vi "GOOP_CreateDefaultIniFile.vi"() -> (1 "NativeRead":path, 2 "NativeWrite":path)   [LabVIEW 2020]
uses:
  <resource>/Framework/Providers/Open_GDS/ClassProviders/Provider_EndevoGOOP300/EndevoProviderName.ctl
  <resource>/Framework/Providers/Open_GDS/ClassProviders/Provider_LvNativeClass/LvNativeProviderName.ctl
  <resource>/Framework/Providers/Open_GDS/ClassProviders/Provider_EndevoGOOP400/EndevoG4ProviderName.ctl
  <vilib>/Utility/config.llb/Write Key (String).vi
  <vilib>/Utility/config.llb/NI_LVConfig.lvlib
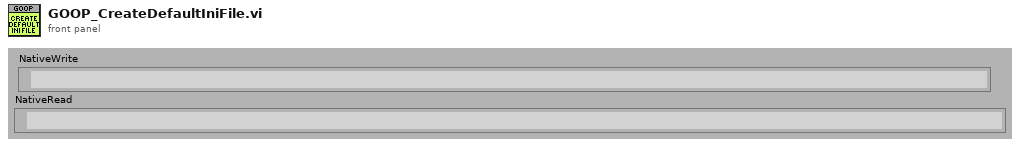
[diagram p1: front panel]
types:
  T1 = typedef "EndevoG4ProviderName.ctl" = enum16{"EndevoGOOP400"}
  T2 = typedef "LvNativeProviderName.ctl" = enum16{"Endevo LabVIEW Native"}
  T3 = typedef "EndevoProviderName.ctl" = enum16{"EndevoGOOP300"}
  T4 = typedef "NI_LVConfig.lvlib/Config Data RefNum.ctl" = refnum<k1>
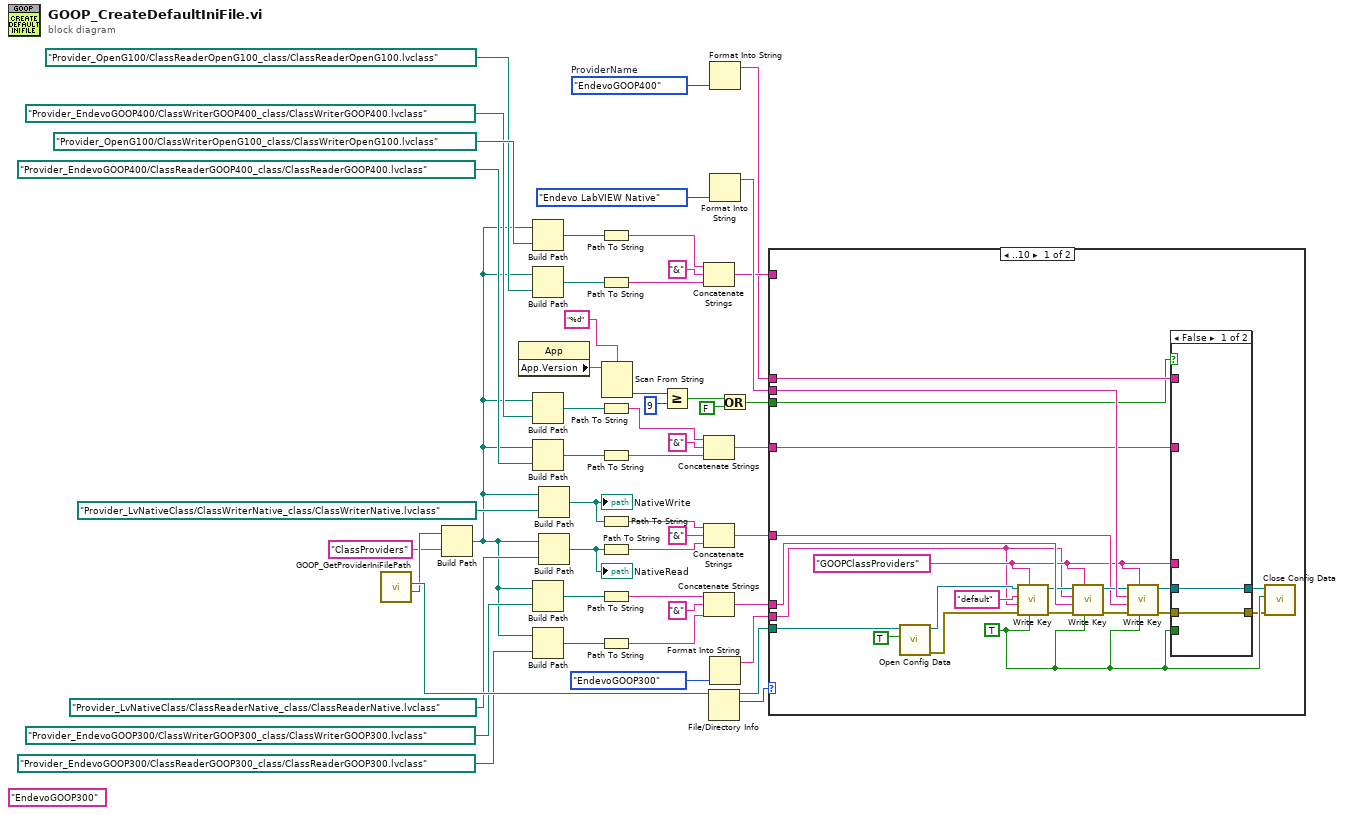
[diagram p0: block diagram]
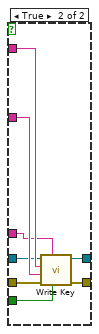
[diagram p2: hidden frame]
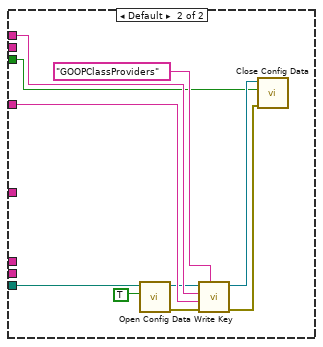
[diagram p3: hidden frame]
diagram:
  w1 = EndevoG4ProviderName."EndevoGOOP400"  # ProviderName
  (unwired) "EndevoGOOP300" ("section")
  n1 = call <resource>:"GOOP_GetProviderIniFilePath.vi"() -> ("ProviderMainFolder"=w20:path, "ProviderIniPath"=w48:path)  [unwired: 10 in]
  n2 = Build Path(base path=w20, name or relative path="ClassProviders") -> (appended path=w15:path)
  n3 = property class="App"() -> ("App.Version"=w13:string)  [unwired: 2 in, 2 out]
  n4 = Build Path(base path=w15, name or relative path=path "Provider_OpenG100/ClassWriterOpenG100_class/ClassWriterOpenG100.lvclass" ("base path")) -> (appended path=w28:path)
  n5 = Build Path(base path=w15, name or relative path=path "Provider_OpenG100/ClassReaderOpenG100_class/ClassReaderOpenG100.lvclass" ("base path")) -> (appended path=w27:path)
  n6 = Build Path(base path=w15, name or relative path=path "Provider_EndevoGOOP400/ClassWriterGOOP400_class/ClassWriterGOOP400.lvclass" ("base path")) -> (appended path=w5:path)
  n7 = Build Path(base path=w15, name or relative path=path "Provider_EndevoGOOP400/ClassReaderGOOP400_class/ClassReaderGOOP400.lvclass" ("base path")) -> (appended path=w6:path)
  n8 = Build Path(base path=w15, name or relative path=path "Provider_EndevoGOOP300/ClassWriterGOOP300_class/ClassWriterGOOP300.lvclass" ("base path")) -> (appended path=w35:path)
  n9 = Build Path(base path=w15, name or relative path=path "Provider_EndevoGOOP300/ClassReaderGOOP300_class/ClassReaderGOOP300.lvclass" ("base path")) -> (appended path=w34:path)
  n10 = Build Path(base path=w15, name or relative path=path "Provider_LvNativeClass/ClassWriterNative_class/ClassWriterNative.lvclass" ("base path")) -> (appended path=w29:path)
  "NativeWrite" <- w29
  n11 = Build Path(base path=w15, name or relative path=path "Provider_LvNativeClass/ClassReaderNative_class/ClassReaderNative.lvclass" ("base path")) -> (appended path=w21:path)
  "NativeRead" <- w21
  n12 = Path To String(path=w28) -> (string=w24:string)
  n13 = Path To String(path=w27) -> (string=w25:string)
  n14 = Path To String(path=w5) -> (string=w9:string)
  n15 = Path To String(path=w6) -> (string=w8:string)
  n16 = Path To String(path=w29) -> (string=w33:string)
  n17 = Path To String(path=w21) -> (string=w32:string)
  n18 = Path To String(path=w35) -> (string=w36:string)
  n19 = Path To String(path=w34) -> (string=w37:string)
  n20 = Scan From String(format string="%d", input string=w13) -> (output 1=w11:i32)  [unwired: 3 in, 3 out]
  n21 = Greater Or Equal?(x=w11, y=9) -> (x >= y?=w4:bool)
  n22 = Concatenate Strings(w24, "&" ("regular expression"), w25) -> (w23:string)
  n23 = Concatenate Strings(w9, "&" ("regular expression"), w8) -> (w18:string)
  n24 = Concatenate Strings(w33, "&" ("regular expression"), w32) -> (w30:string)
  n25 = Concatenate Strings(w36, "&" ("regular expression"), w37) -> (w39:string)
  n26 = File/Directory Info(path=w48) -> (path out=w51:path, size=w22:i64)  [unwired: 1 in, 5 out]
  n27 = Format Into String(w1) -> (resulting string=w14:string)  [unwired: 3 in, 1 out]
  n28 = Format Into String(LvNativeProviderName."Endevo LabVIEW Native" ("ProviderName")) -> (resulting string=w40:string)  [unwired: 3 in, 1 out]
  n29 = Format Into String(EndevoProviderName."EndevoGOOP300" ("ProviderName")) -> (resulting string=w49:string)  [unwired: 3 in, 1 out]
  n30 = Or(x=w4, y=FALSE) -> (x .or. y?=w3:bool)
  n31 = case shown="..10" w22 {
    tunnel: w51 -> [w73 w93]
    tunnel: w49 -> [w52 _]
    tunnel: w40 -> [w72 _]
    tunnel: w39 -> [w67 _]
    tunnel: w30 -> [w62 _]
    tunnel: w23 -> [_ _]
    tunnel: w14 -> [w60 w90]
    tunnel: w18 -> [w61 w91]
    tunnel: w3 -> [w55 w84]
    frame ..10 {
      w56 = TRUE ("write configuration file? (T)")
      w57 = "GOOPClassProviders" ("section")
      n32 = call <vilib>:"Open Config Data.vi"("create file if necessary (T)"=TRUE ("create file if necessary? (T)"), "configuration file path"=w73) -> ("error out"=w69:errorcluster, "refnum"=w68:T4)  [unwired: 7 in, 1 out]
      n33 = call-poly <vilib>:"Write Key.vi"("write raw string? (F)"=w56, "section"=w57, "error in (no error)"=w69, "value"=w52, "key"="default", "refnum"=w68) -> ("error out"=w66:errorcluster, "refnum out"=w65:T4)  [unwired: 3 in, 1 out]
      n34 = call-poly <vilib>:"Write Key.vi"("write raw string? (F)"=w56, "section"=w57, "error in (no error)"=w66, "value"=w67, "key"=w52, "refnum"=w65) -> ("error out"=w64:errorcluster, "refnum out"=w63:T4)  [unwired: 3 in, 1 out]
      n35 = call-poly <vilib>:"Write Key.vi"("write raw string? (F)"=w56, "section"=w57, "error in (no error)"=w64, "value"=w62, "key"=w72, "refnum"=w63) -> ("error out"=w58:errorcluster, "refnum out"=w59:T4)  [unwired: 3 in, 1 out]
      n36 = case shown="False" w55 {
        tunnel: w61 -> [_ w83]
        tunnel: w60 -> [_ w82]
        tunnel: w59 -> [w75 w81]
        tunnel: w58 -> [w74 w80]
        tunnel: [w74 w79] -> w54
        tunnel: [w75 w78] -> w53
        tunnel: w57 -> [_ w77]
        tunnel: w56 -> [_ w76]
        frame False {
        }
        frame True {
          n37 = call-poly <vilib>:"Write Key.vi"("write raw string? (F)"=w76, "section"=w77, "error in (no error)"=w80, "value"=w83, "key"=w82, "refnum"=w81) -> ("error out"=w79:errorcluster, "refnum out"=w78:T4)  [unwired: 3 in, 1 out]
        }
      }
      n38 = call <vilib>:"Close Config Data.vi"("error in (no error)"=w54, "write file if changed (T)"=w56, "refnum"=w53) -> ()  [unwired: 7 in, 2 out]
    }
    frame Default {
      n39 = call <vilib>:"Open Config Data.vi"("create file if necessary (T)"=TRUE ("create file if necessary? (T)"), "configuration file path"=w93) -> ("error out"=w87:errorcluster, "refnum"=w88:T4)  [unwired: 7 in, 1 out]
      n40 = call-poly <vilib>:"Write Key.vi"("section"="GOOPClassProviders", "error in (no error)"=w87, "value"=w91, "key"=w90, "refnum"=w88) -> ("error out"=w85:errorcluster, "refnum out"=w86:T4)  [unwired: 4 in, 1 out]
      n41 = call <vilib>:"Close Config Data.vi"("error in (no error)"=w85, "write file if changed (T)"=w84, "refnum"=w86) -> ()  [unwired: 7 in, 2 out]
    }
  }
